vi "Serial read all.vi"(6 "timeout (10000ms)":u32=10000, 8 "error in (no error)":errorcluster, 9 "Wait for OK":bool, 11 "VISA Refnum in":refnum<visa-resource-name>) -> (0 "error out":errorcluster, 1 "command OK":bool, 2 "read buffer":string, 3 "VISA Refnum out":refnum<visa-resource-name>)   [LabVIEW 2023, in "Marlin Instrument Driver.lvlib"]
uses:
  Marlin Instrument Driver.lvlib
  <vilib>/Utility/error.llb/Trim Whitespace One-Sided.vi
  <vilib>/Utility/error.llb/Error Cluster From Error Code.vi
  <vilib>/ErrorRing/Error Ring.xnode
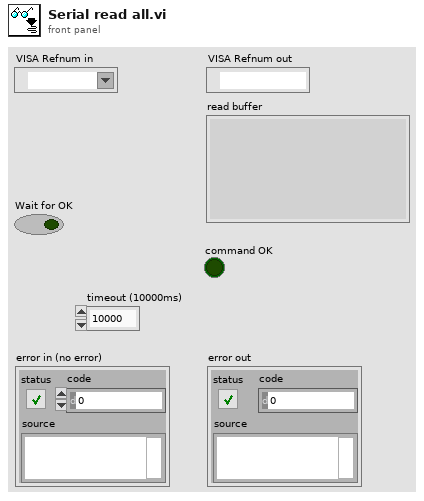
[diagram p1: front panel]
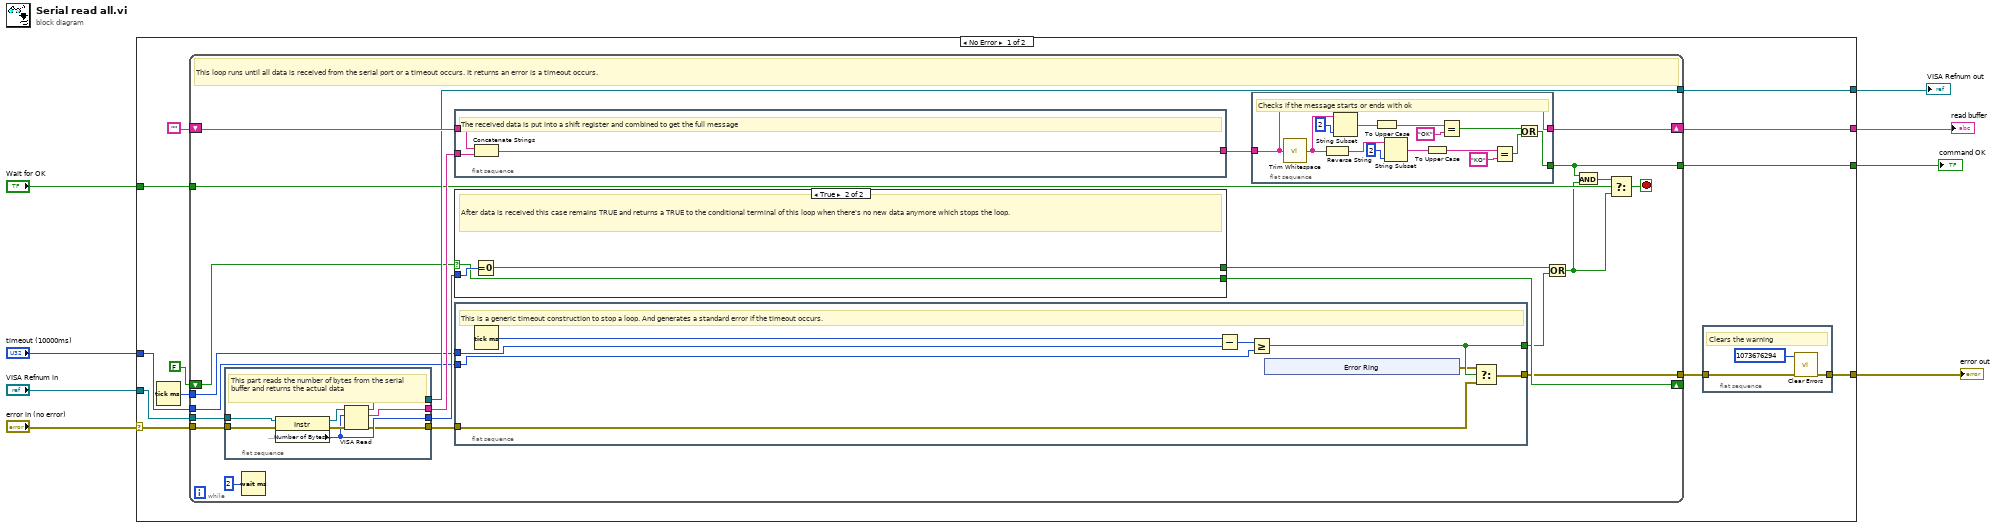
[diagram p0: block diagram]
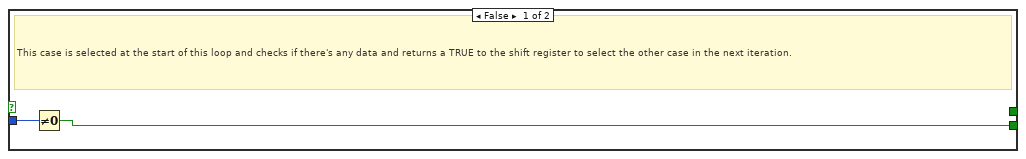
[diagram p2: hidden frame]
diagram:
  n1 = case shown="No Error" "error in (no error)" {
    selector: "error in (no error)" -> [w11 w89]
    tunnel: "timeout (10000ms)" -> [w20 _]
    tunnel: [w17 w88] -> w7
    tunnel: [w14 w89] -> w6
    tunnel: [w13 _] -> w5
    tunnel: "Wait for OK" -> [w12 _]
    tunnel: "VISA Refnum in" -> [w10 w88]
    tunnel: [w9 _] -> w1
    frame No Error {
      n2 = Tick Count (ms)() -> (millisecond timer value=w19:u32)
      n3 = while {
        tunnel: w10 -> [w44]
        tunnel: w11 -> [w43]
        shift-right: [w31] -> w13
        shift-left: "" -> [w42]
        tunnel: [w33] -> w15
        tunnel: [w40] -> w17
        shift-right: [w38] -> _
        shift-left: FALSE -> [w37]
        tunnel: w19 -> [w36]
        tunnel: w20 -> [w35]
        tunnel: w12 -> [w30]
        tunnel: [w26] -> w9
        stop <- w29 stop-if-true
        # "This loop runs until all data is received from the serial port or a timeout occurs. It returns an error is a timeout occurs."
        n4 = flat-sequence {
          tunnel: w44 -> [w82]
          tunnel: w43 -> [w81]
          tunnel: [w78] -> w41
          tunnel: [w77] -> w40
          tunnel: [w76] -> w39
          tunnel: [w75] -> w34
          frame #0 {
            # "This part reads the number of bytes from the serial buffer and returns the actual data"
            n5 = property class="Instr"(reference=w82, error in=w81) -> (reference out=w80:refnum<visa-resource-name>, error out=w79:errorcluster, "Serial Settings:Number of Bytes at Serial Port"=w76:u32)
            n6 = VISA Read(VISA resource name=w80, byte count=w76, error in (no error)=w79) -> (VISA resource name out=w77:refnum<visa-resource-name>, read buffer=w78:string, error out=w75:errorcluster)  [unwired: 1 out]
          }
        }
        n7 = Wait (ms)(milliseconds to wait=u32 2) -> ()  [unwired: 1 out]
        n8 = flat-sequence {
          tunnel: w42 -> [w62]
          tunnel: w41 -> [w61]
          tunnel: [w60] -> w32
          frame #0 {
            # "The received data is put into a shift register and combined to get the full message"
            n9 = Concatenate Strings(w62, w61) -> (w60:string)
          }
        }
        n10 = case shown="True" w37 {
          selector: w37 -> [_ w85]
          tunnel: w39 -> [w84 w87]
          tunnel: [w83 w85] -> w38
          tunnel: [_ w86] -> w24
          frame False {
            # "This case is selected at the start of this loop and checks if there's any data and returns a TRUE to the shift register to select the other case in the next iteration."
            n11 = Not Equal To 0?(x=w84) -> (x != 0?=w83:bool)
          }
          frame True {
            # "After data is received this case remains TRUE and returns a TRUE to the conditional terminal of this loop when there's no new data anymore which stops the loop."
            n12 = Equal To 0?(x=w87) -> (x = 0?=w86:bool)
          }
        }
        n13 = flat-sequence {
          tunnel: w36 -> [w69]
          tunnel: w35 -> [w67]
          tunnel: [w66] -> w25
          tunnel: w34 -> [w64]
          tunnel: [w63] -> w33
          frame #0 {
            # "This is a generic timeout construction to stop a loop. And generates a standard error if the timeout occurs."
            n14 = Tick Count (ms)() -> (millisecond timer value=w70:u32)
            n15 = Subtract(x=w70, y=w69) -> (x-y=w68:u32)
            n16 = Greater Or Equal?(x=w68, y=w67) -> (x >= y?=w66:bool)
            n17 = xnode "Error Ring"() -> ("error out"=w65:errorcluster)
            n18 = Select(t=w65, s=w66, f=w64) -> (s? t:f=w63:errorcluster)
          }
        }
        n19 = flat-sequence {
          tunnel: [w46] -> w26
          tunnel: w32 -> [w52]
          tunnel: [w52] -> w31
          frame #0 {
            # "Checks if the message starts or ends with ok"
            n20 = call <vilib>:"Trim Whitespace.vi"("string"=w52) -> ("trimmed string"=w48:string)  [unwired: 1 in]
            n21 = Reverse String(1:w48) -> (0:w59:string)
            n22 = String Subset(string=w48, length (rest)=2 ("length (rest)")) -> (substring=w53:string)  [unwired: 1 in]
            n23 = To Upper Case(1:w53) -> (0:w50:string)
            n24 = String Subset(string=w59, length (rest)=2 ("length (rest)")) -> (substring=w57:string)  [unwired: 1 in]
            n25 = To Upper Case(1:w57) -> (0:w56:string)
            n26 = Equal?(x=w50, y="OK") -> (x = y?=w49:bool)
            n27 = Equal?(x=w56, y="KO") -> (x = y?=w47:bool)
            n28 = Or(x=w49, y=w47) -> (x .or. y?=w46:bool)
          }
        }
        n29 = Or(x=w24, y=w25) -> (x .or. y?=w28:bool)
        n30 = And(x=w26, y=w28) -> (x .and. y?=w27:bool)
        n31 = Select(t=w27, s=w30, f=w28) -> (s? t:f=w29:bool)
      }
      n32 = flat-sequence {
        tunnel: w15 -> [w22]
        tunnel: [w21] -> w14
        frame #0 {
          # "Clears the warning"
          n33 = call <vilib>:"Clear Errors.vi"("error in (no error)"=w22, "specific error code to clear (0: all)"=1073676294) -> ("error out"=w21:errorcluster)  [unwired: 4 in, 1 out]
        }
      }
    }
    frame Error {
      # "This VI is skipped when an error occurs and the error is passed through"
    }
  }
  "VISA Refnum out" <- w7
  "read buffer" <- w5
  "error out" <- w6
  "command OK" <- w1
